vi "Digital Offset.vi"(0 "data in":T1[](array[typedef])=[{"I"=0.0, "Q"=0.0, "overflow"=FALSE}, {"I"=0.0, "Q"=0.0, "overflow"=FALSE}], 9 "input valid":bool, 11 "gen in":refnum<class "niUSRP Tx DSP v2 FPGA.lvclass">, 12 "ready for output (T)":bool=TRUE) -> (4 "data out":T1[](array[typedef]), 10 "output valid":bool, 14 "ready for input":bool, 15 "gen out":refnum<class "niUSRP Tx DSP v2 FPGA.lvclass">)   [LabVIEW 2025, in "niUSRP Tx DSP v2 FPGA.lvclass"]
uses:
  niUSRP Tx DSP v2 FPGA.lvclass
  <instrlib>/_niInstr/DSP/v1/Shared/Public/IQ Data.ctl
  <instrlib>/_niInstr/DSP Control/Interface/v1/FPGA/Digital Offset/IQ 18-bit/Digital Offset Interface (IQ 18-bit).lvclass
  <instrlib>/_niInstr/Basic Elements/v1/FPGA/niInstr Basic Elements v1 FPGA.lvlib
  <instrlib>/_niInstr/DSP/v1/Shared/niInstr DSP v1 Shared.lvlib
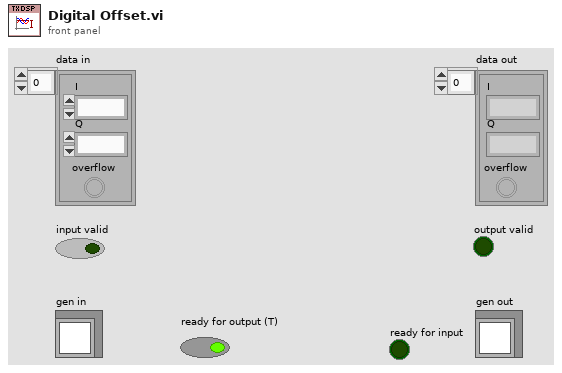
[diagram p1: front panel]
types:
  T1 = typedef "niInstr DSP v1 Shared.lvlib/IQ Data.ctl" = cluster{"I":fxp<+/-,18,1>, "Q":fxp<+/-,18,1>, "overflow":bool}
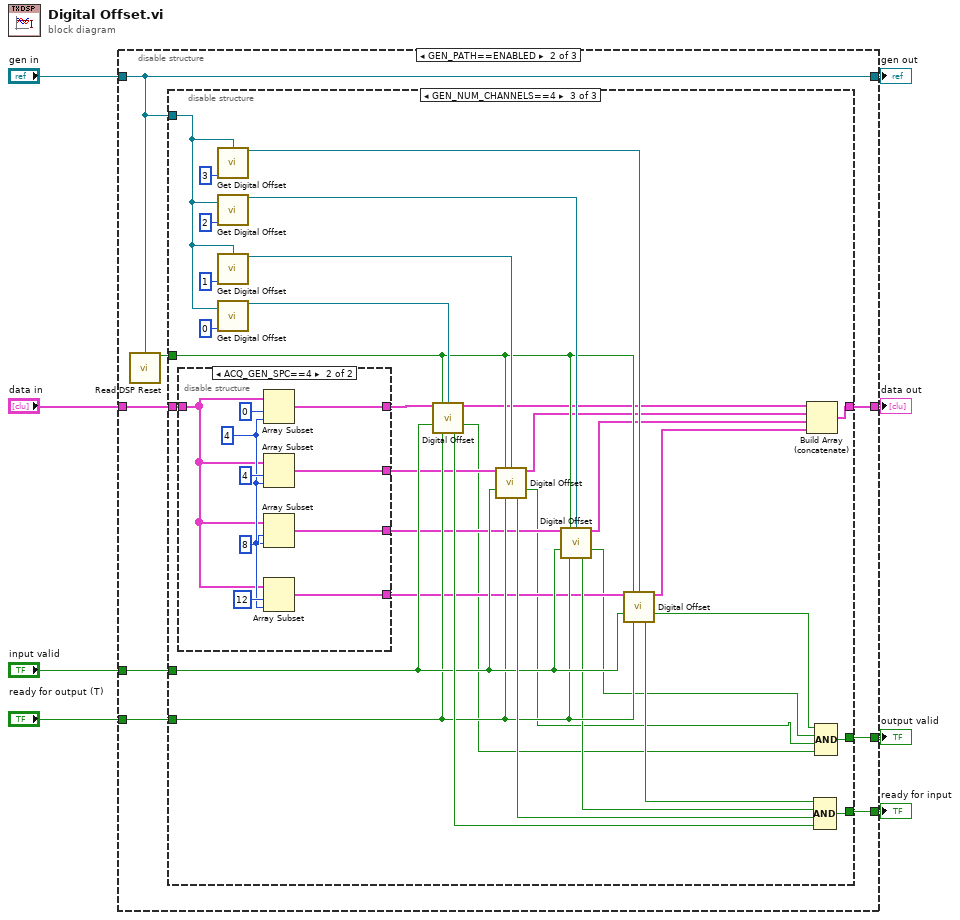
[diagram p0: block diagram]
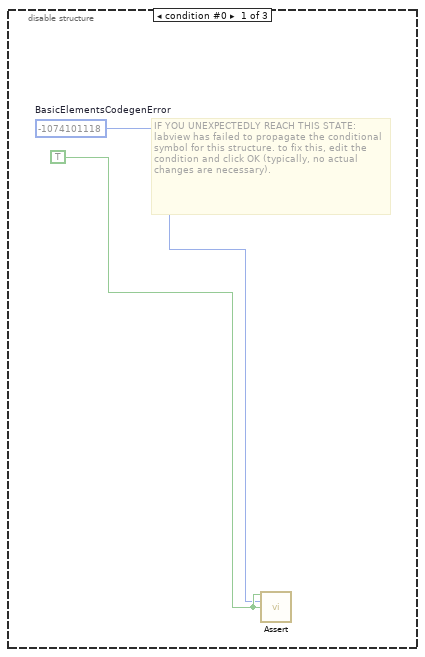
[diagram p2: hidden frame]
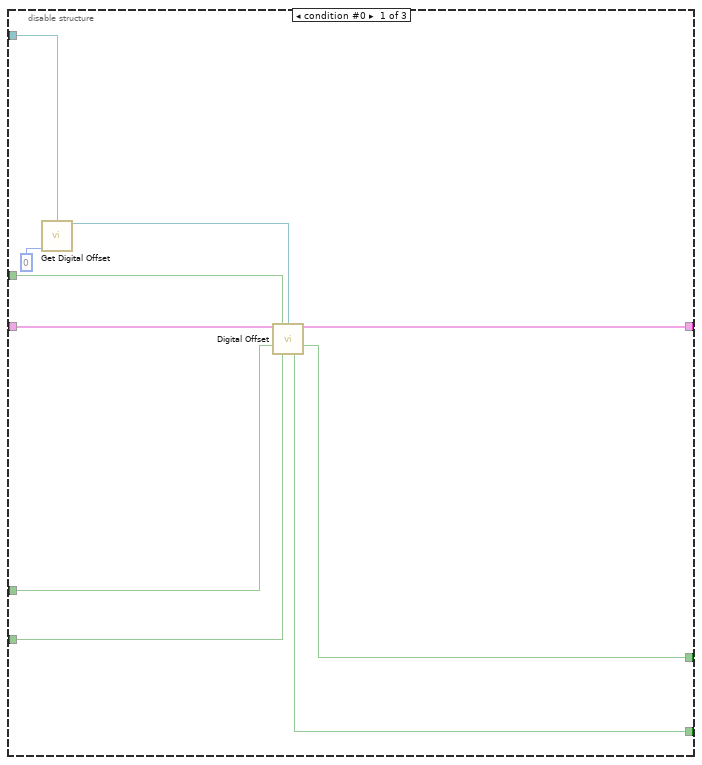
[diagram p3: hidden frame]
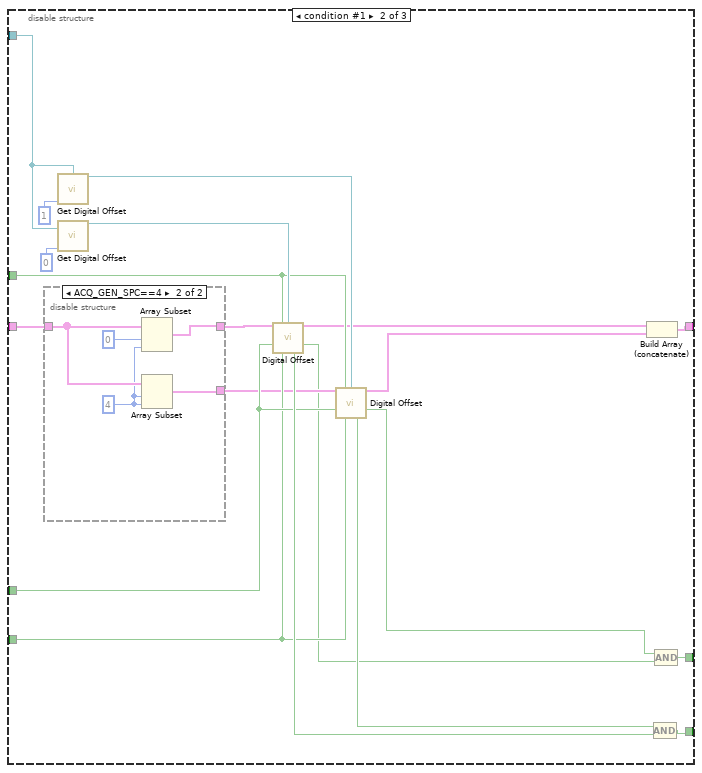
[diagram p4: hidden frame]
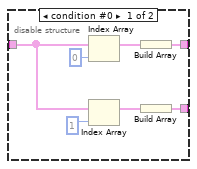
[diagram p5: hidden frame]
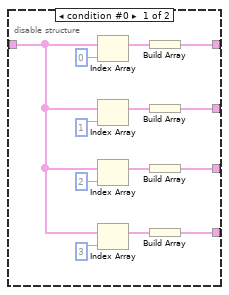
[diagram p6: hidden frame]
diagram:
  n1 = disable-structure shown="GEN_PATH==ENABLED" {
    disable-tunnel: "input valid" -> [_ w18 w116]
    disable-tunnel: "ready for output (T)" -> [_ w17 w117]
    disable-tunnel: [_ w16 w116] -> w6
    disable-tunnel: "gen in" -> [_ w11 w119]
    disable-tunnel: [_ w11 w119] -> w5
    disable-tunnel: "data in" -> [_ w15 w118]
    disable-tunnel: [_ w14 w118] -> w3
    disable-tunnel: [_ w12 w117] -> w2
    frame condition #0 {
      w10 = TRUE ("assert")
      w9 = -1074101118  # BasicElementsCodegenError
      # "IF YOU UNEXPECTEDLY REACH THIS STATE:\nlabview has failed to propagate the conditional symbol for this structure. to fix this, edit the condition and click OK (typically, no actual changes are necessary)."
      n2 = call <instrlib>:"Assert.vi"("assert"=w10, "error code"=w9, "enable show error"=w10) -> ()  [unwired: 13 in]
    }
    frame condition #1 (active) {
      n3 = call-dynamic "Read DSP Reset.vi"("gen"=w11) -> ("dsp reset"=w13:bool)  [unwired: 14 in]
      n4 = disable-structure shown="GEN_NUM_CHANNELS==4" {
        disable-tunnel: w18 -> [w28 w42 w77]
        disable-tunnel: w17 -> [w27 w41 w76]
        disable-tunnel: [w26 w46 w90] -> w16
        disable-tunnel: w15 -> [w25 w35 w73]
        disable-tunnel: [w24 w47 w91] -> w14
        disable-tunnel: w13 -> [w23 w43 w78]
        disable-tunnel: [w22 w44 w88] -> w12
        disable-tunnel: w11 -> [w20 w39 w81]
        frame condition #0 {
          n5 = call-dynamic "Get Digital Offset.vi"("gen"=w20, "ch"=u8 0) -> ("digital offset"=w21:refnum<class "Digital Offset Interface (IQ 18-bit).lvclass">)  [unwired: 13 in]
          n6 = call-dynamic "Digital Offset.vi"("data in"=w25, "reset"=w23, "digital offset"=w21, "input valid"=w28, "ready for output (T)"=w27) -> ("data out"=w24:T1[], "output valid"=w26:bool, "ready for input"=w22:bool)  [unwired: 7 in, 1 out]
        }
        frame condition #1 {
          n7 = disable-structure shown="ACQ_GEN_SPC==4" {
            disable-tunnel: w35 -> [w51 w58]
            disable-tunnel: [w50 w59] -> w34
            disable-tunnel: [w49 w57] -> w33
            frame condition #0 {
              n8 = Index Array(array=w51, index=0) -> (element=w55:T1)
              n9 = Index Array(array=w51, index=1) -> (element=w53:T1)
              n10 = Build Array(w55) -> (w50:T1[])
              n11 = Build Array(w53) -> (w49:T1[])
            }
            frame condition #1 (active) {
              w56 = 4 ("length")
              n12 = Array Subset(array=w58, index=0, length=w56) -> (w59:T1[])
              n13 = Array Subset(array=w58, index=w56, length=w56) -> (w57:T1[])
            }
          }
          n14 = call-dynamic "Get Digital Offset.vi"("gen"=w39, "ch"=u8 1) -> ("digital offset"=w38:refnum<class "Digital Offset Interface (IQ 18-bit).lvclass">)  [unwired: 13 in]
          n15 = call-dynamic "Get Digital Offset.vi"("gen"=w39, "ch"=u8 0) -> ("digital offset"=w48:refnum<class "Digital Offset Interface (IQ 18-bit).lvclass">)  [unwired: 13 in]
          n16 = call-dynamic "Digital Offset.vi"("data in"=w34, "reset"=w43, "digital offset"=w48, "input valid"=w42, "ready for output (T)"=w41) -> ("data out"=w32:T1[], "output valid"=w29:bool, "ready for input"=w45:bool)  [unwired: 7 in, 1 out]
          n17 = call-dynamic "Digital Offset.vi"("data in"=w33, "reset"=w43, "digital offset"=w38, "input valid"=w42, "ready for output (T)"=w41) -> ("data out"=w31:T1[], "output valid"=w30:bool, "ready for input"=w40:bool)  [unwired: 7 in, 1 out]
          n18 = Build Array (concatenate)(w32, w31) -> (w47:T1[])
          n19 = Compound Arithmetic op=AND(w40, w45) -> (w44:bool)
          n20 = Compound Arithmetic op=AND(w30, w29) -> (w46:bool)
        }
        frame condition #2 (active) {
          n21 = disable-structure shown="ACQ_GEN_SPC==4" {
            disable-tunnel: [w101 w109] -> w72
            disable-tunnel: [w100 w108] -> w71
            disable-tunnel: [w99 w107] -> w70
            disable-tunnel: w73 -> [w94 w110]
            disable-tunnel: [w93 w106] -> w69
            frame condition #0 {
              n22 = Index Array(array=w94, index=0) -> (element=w105:T1)
              n23 = Index Array(array=w94, index=1) -> (element=w103:T1)
              n24 = Index Array(array=w94, index=2) -> (element=w95:T1)
              n25 = Index Array(array=w94, index=3) -> (element=w97:T1)
              n26 = Build Array(w105) -> (w101:T1[])
              n27 = Build Array(w103) -> (w100:T1[])
              n28 = Build Array(w95) -> (w99:T1[])
              n29 = Build Array(w97) -> (w93:T1[])
            }
            frame condition #1 (active) {
              w111 = 4 ("length")
              n30 = Array Subset(array=w110, index=0, length=w111) -> (w109:T1[])
              n31 = Array Subset(array=w110, index=4, length=w111) -> (w108:T1[])
              n32 = Array Subset(array=w110, index=8, length=w111) -> (w107:T1[])
              n33 = Array Subset(array=w110, index=12, length=w111) -> (w106:T1[])
            }
          }
          n34 = call-dynamic "Get Digital Offset.vi"("gen"=w81, "ch"=u8 3) -> ("digital offset"=w79:refnum<class "Digital Offset Interface (IQ 18-bit).lvclass">)  [unwired: 13 in]
          n35 = call-dynamic "Get Digital Offset.vi"("gen"=w81, "ch"=u8 2) -> ("digital offset"=w80:refnum<class "Digital Offset Interface (IQ 18-bit).lvclass">)  [unwired: 13 in]
          n36 = call-dynamic "Get Digital Offset.vi"("gen"=w81, "ch"=u8 1) -> ("digital offset"=w86:refnum<class "Digital Offset Interface (IQ 18-bit).lvclass">)  [unwired: 13 in]
          n37 = call-dynamic "Get Digital Offset.vi"("gen"=w81, "ch"=u8 0) -> ("digital offset"=w92:refnum<class "Digital Offset Interface (IQ 18-bit).lvclass">)  [unwired: 13 in]
          n38 = call-dynamic "Digital Offset.vi"("data in"=w72, "reset"=w78, "digital offset"=w92, "input valid"=w77, "ready for output (T)"=w76) -> ("data out"=w68:T1[], "output valid"=w61:bool, "ready for input"=w89:bool)  [unwired: 7 in, 1 out]
          n39 = call-dynamic "Digital Offset.vi"("data in"=w71, "reset"=w78, "digital offset"=w86, "input valid"=w77, "ready for output (T)"=w76) -> ("data out"=w67:T1[], "output valid"=w62:bool, "ready for input"=w87:bool)  [unwired: 7 in, 1 out]
          n40 = call-dynamic "Digital Offset.vi"("data in"=w70, "reset"=w78, "digital offset"=w80, "input valid"=w77, "ready for output (T)"=w76) -> ("data out"=w66:T1[], "output valid"=w63:bool, "ready for input"=w75:bool)  [unwired: 7 in, 1 out]
          n41 = call-dynamic "Digital Offset.vi"("data in"=w69, "reset"=w78, "digital offset"=w79, "input valid"=w77, "ready for output (T)"=w76) -> ("data out"=w65:T1[], "output valid"=w64:bool, "ready for input"=w74:bool)  [unwired: 7 in, 1 out]
          n42 = Build Array (concatenate)(w68, w67, w66, w65) -> (w91:T1[])
          n43 = Compound Arithmetic op=AND(w74, w75, w87, w89) -> (w88:bool)
          n44 = Compound Arithmetic op=AND(w64, w63, w62, w61) -> (w90:bool)
        }
      }
    }
    frame condition #2 {
    }
  }
  "data out" <- w3
  "output valid" <- w6
  "ready for input" <- w2
  "gen out" <- w5
